vi "HandleSetParamterErrors.vi"(7 "SetParameter":T1, 8 "error in (no error)":errorcluster, 11 "Phase":i32) -> (0 "error IO":errorcluster, 2 "Status Update":string)   [LabVIEW 2018, in "AcPwrPlugins.lvlib" / "AcPwrBase.lvclass"]
uses:
  AcPwrBase.lvclass
  TypeDefs/SetParameterInputs.ctl
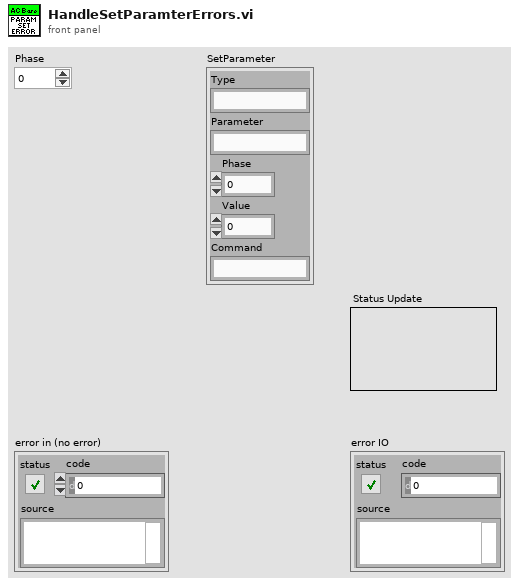
[diagram p1: front panel]
types:
  T1 = typedef "AcPwrPlugins.lvlib/AcPwrBase.lvclass/SetParameterInputs.ctl" = cluster{"Type":string, "Parameter":string, "Phase":i32, "Value":dbl, "Command":string}
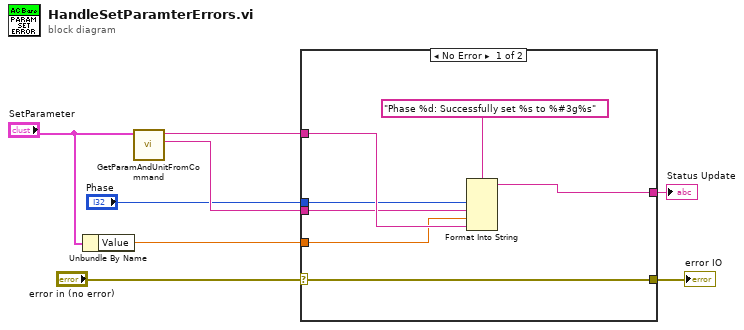
[diagram p0: block diagram]
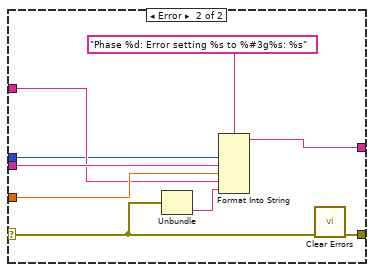
[diagram p2: hidden frame]
diagram:
  n1 = Unbundle By Name("SetParameter") -> ("Value"=w2:dbl)
  n2 = call "GetParamAndUnitFromCommand.vi"("SetParameter"="SetParameter") -> ("Parameter"=w4:string, "Unit Label"=w6:string)  [unwired: 9 in]
  n3 = case shown="No Error" "error in (no error)" {
    selector: "error in (no error)" -> [w10 w22]
    tunnel: w4 -> [w13 w24]
    tunnel: [w10 w21] -> w7
    tunnel: w6 -> [w14 w19]
    tunnel: w2 -> [w12 w20]
    tunnel: [w11 w17] -> w5
    tunnel: "Phase" -> [w9 w16]
    frame No Error {
      n4 = Format Into String(format string="Phase %d: Successfully set %s to %#3g%s", w9, w13, w12, w14) -> (resulting string=w11:string)  [unwired: 2 in, 1 out]
    }
    frame Error {
      n5 = Unbundle(w22) -> ("source"=w18:string)  [unwired: 2 out]
      n6 = Format Into String(format string="Phase %d: Error setting %s to %#3g%s: %s" ("Handle"), w16, w24, w20, w19, w18) -> (resulting string=w17:string)  [unwired: 2 in, 1 out]
      n7 = call <vilib>:"Clear Errors.vi"("error in (no error)"=w22) -> ("error out"=w21:errorcluster)  [unwired: 5 in, 1 out]
    }
  }
  "error IO" <- w7
  "Status Update" <- w5
